vi "ATF-CS signal names FGV.vi"(7 "Enum":enum16{"Read", "Write"}(ring), 8 "error in":errorcluster, 11 "Signal names":T1) -> (0 "error out":errorcluster, 3 "Signal names R":T1)   [LabVIEW 2022 SP3]
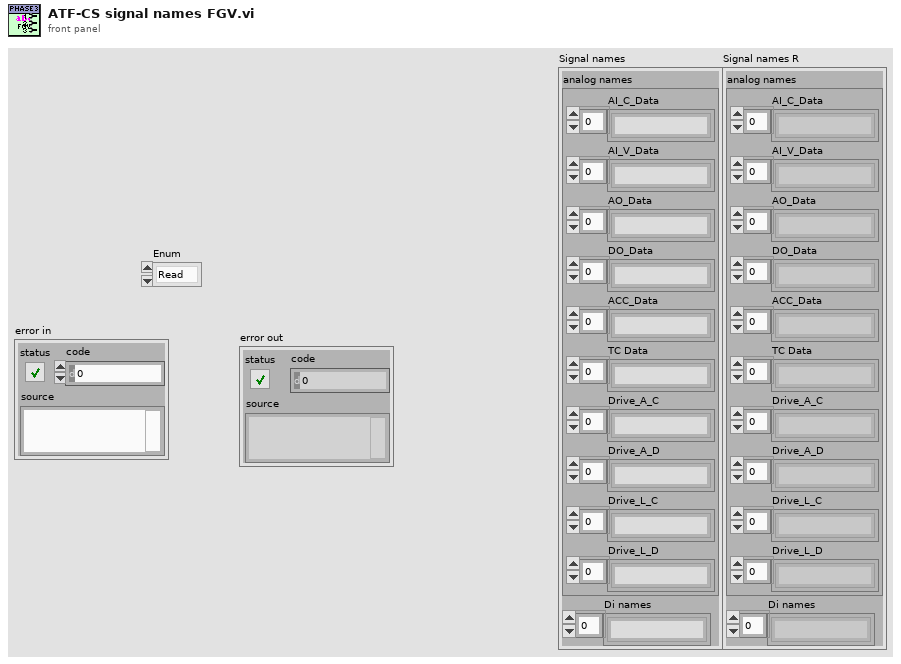
[diagram p1: front panel]
types:
  T1 = cluster{"analog names":cluster{"AI_C_Data":string[], "AI_V_Data":string[], "AO_Data":string[], "DO_Data":string[], "ACC_Data":string[], "TC Data":string[], "Drive_A_C":string[], "Drive_A_D":string[], "Drive_L_C":string[], "Drive_L_D":string[]}, "Di names":string[]}
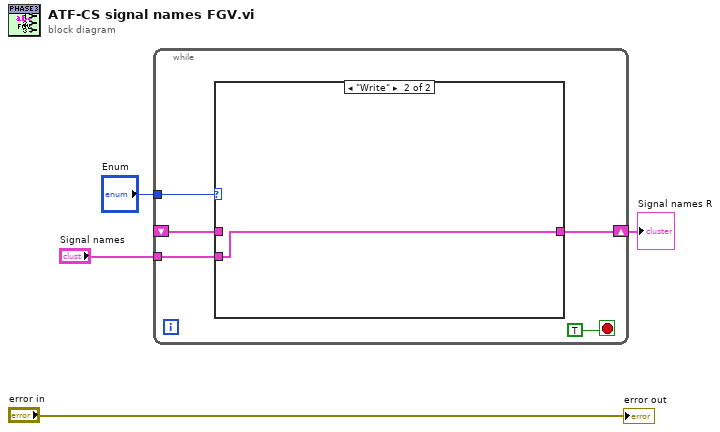
[diagram p0: block diagram]
diagram:
  n1 = while {
    tunnel: "Enum" -> [w9]
    tunnel: "Signal names" -> [w7]
    shift-right: [w6] -> w1
    shift-left: _ -> [w5]
    stop <- TRUE stop-if-true
    n2 = case shown="\"Write\"" w9 {
      tunnel: w7 -> [_ w11]
      tunnel: [w10 w11] -> w6
      tunnel: w5 -> [w10 _]
      frame "Read", Default {
      }
      frame "Write" {
      }
    }
  }
  "Signal names R" <- w1
  "error out" <- "error in"
